vi "Autonomous Independent.vi"() -> ()   [LabVIEW 2017]
doc: "This VI is called when autonomous begins, and will automatically be terminated when autonomous ends. You can carry out timed or sensor driven robot movement independently without needing to return to the caller."
uses:
  <vilib>/Rock Robotics/WPI/DriverStation/WPI_DriverStationPositionInfo.ctl
  <vilib>/Rock Robotics/WPI/DriverStation/WPI_DriverStationAllianceInfo.ctl
  Public/Documents/Cross The Road Electronics/Phoenix-LabVIEW/Motor Controller/Controls/CTRE_Phoenix_MotorControl_ControlMode.ctl
  <vilib>/Rock Robotics/Network Tables/NT Read String.vi
  <vilib>/Rock Robotics/Network Tables/NT Read Number.vi
  <vilib>/Rock Robotics/Network Tables/NT Read Numeric Array.vi
  <vilib>/Rock Robotics/Network Tables/NT Read String Array.vi
  Robot Global Data.vi
  <vilib>/Rock Robotics/WPI/Ultrasonic/WPI_SonarMB1010AnalogRefNum Registry Get.vi
  <vilib>/Rock Robotics/WPI/Ultrasonic/WPI_SonarMB1010AnalogGetRange.vi
panel:
  out "Alliance":T1
  out "Position":T2
  out "FMS Data Array":string[](array[string])
  out "Scale":string
  out "Switch":string
  out "Setpoint2":dbl
  out "Setpoint":dbl
  in  "Z Drive PID Gains":T3={"Position"=0.04, "Interval"=0.0, "Derivative"=0.0}
  # "Be sure to right-click and choose Data Operations>>Make Current Value default if you want to save the array values with the VI"
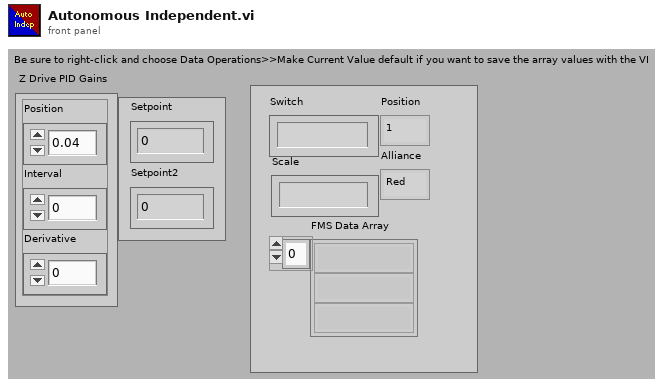
[diagram p1: front panel]
types:
  T1 = typedef "WPI_DriverStationAllianceInfo.ctl" = enum16{"Red", "Blue", "Invalid"}
  T2 = typedef "WPI_DriverStationPositionInfo.ctl" = enum16{"1", "2", "3"}
  T3 = cluster{"Position":dbl, "Interval":dbl, "Derivative":dbl}
  T4 = enum16{"Front Left", "Front Right", "Back Left", "Back Right"}
  T5 = typedef "WPI_SonarMB1010AnalogDeviceRef.ctl" = cluster{"AIDeviceRef":T6, "Scaling factor (V/in)":dbl, "Average Bits":u8}
  T6 = typedef "WPI_AnalogChannelDevRef.ctl" = cluster{"DevStatus":errorcluster, "Analog Channel":T7}
  T7 = typedef "FPGA_AIChannel.ctl" = enum8{"AI 0", "AI 1", "AI 2", "AI 3", "AI MXP 0", "AI MXP 1", "AI MXP 2", "AI MXP 3", "Invalid"}
  T8 = typedef "WPI_AccelerometerDevRef.ctl" = cluster{"DevStatus":errorcluster, "Scaling":T9, "Analog Channels":T10, "I2C Bus":T11, "SPI Bus":T12, "Accel Range":T13, "ADXL Axes":T14, "Handle":i32, "Device Address":u8, "Accel Type":enum16{"Analog", "ADXL345 I2C", "ADXL345 SPI", "Internal", "ADXL362 SPI"}}
  T9 = typedef "WPI_AccelerometerScaling.ctl" = cluster{"Gain (VoltsPerG)":dbl, "Center Voltage":dbl}
  T10 = typedef "WPI_AccelerometerAnalogChannels.ctl" = cluster{"X-Axis":T7, "Y-Axis":T7, "Z-Axis":T7}
  T11 = typedef "i2c_bus.ctl" = enum16{"I2C On-Board", "I2C MXP", "Invalid"}
  T12 = typedef "spi_bus.ctl" = enum16{"SPI On-Board, CS0", "SPI On-Board, CS1", "SPI On-Board, CS2", "SPI On-Board, CS3", "SPI MXP", "Invalid"}
  T13 = typedef "ADXL345 Range.ctl" = u8
  T14 = typedef "WPI_AccelerometerADXL345 Axes.ctl" = cluster{"X-Axis":bool, "Y-Axis":bool, "Z-Axis":bool}
  T15 = cluster{"X-Axis":dbl, "Y-Axis":dbl, "Z-Axis":dbl}
  T16 = typedef "WPI_EncoderDevRef.ctl" = cluster{"DevStatus":errorcluster, "EncoderIndex":T17, "CounterIndex":T18, "DistancePerCount":dbl, "Decoding Type":T19}
  T17 = typedef "FPGA_EncoderIdx.ctl" = enum8{"Enc 0", "Enc 1", "Enc 2", "Enc 3", "Enc 4", "Enc 5", "Enc 6", "Enc 7", "Invalid"}
  T18 = typedef "FPGA_CounterCtrSystemIndex.ctl" = enum8{"Ctr 0", "Ctr 1", "Ctr 2", "Ctr 3", "Ctr 4", "Ctr 5", "Ctr 6", "Ctr 7", "Invalid"}
  T19 = typedef "WPI_EncoderType.ctl" = enum16{"1x", "2x", "4x"}
  T20 = typedef "WPI_MotorControlDeviceRef.ctl" = cluster{"DeviceStatus":errorcluster, "Type":T21, "PWM":cluster{"PWM Channel":T22, "DeadBand":T23}, "CAN":cluster{"Device Number":u8, "SetOutput VI Ref":variant, "GetOutput VI Ref":variant, "Enable VI Ref":variant, "Disable VI Ref":variant, "Data":variant}, "Invert":bool, "DIO PWM":cluster{"PWM \"Enable\" Channel":T22, "DIOChannel":T24, "PWM Rate":dbl}}
  T21 = typedef "WPI_MotorControlType.ctl" = enum16{"PWM", "CAN", "DIO PWM"}
  T22 = typedef "FPGA_DIOPWMChannel.ctl" = enum8{"PWM 0", "PWM 1", "PWM 2", "PWM 3", "PWM 4", "PWM 5", "PWM 6", "PWM 7", "PWM 8", "PWM 9", "PWM MXP 0", "PWM MXP 1", "PWM MXP 2", "PWM MXP 3", "PWM MXP 4", "PWM MXP 5", "PWM MXP 6", "PWM MXP 7", "PWM MXP 8", "PWM MXP 9", "Invalid"}
  T23 = typedef "WPI_PWMDeadband.ctl" = cluster{"Name":string, "maxPositivePwm":i32, "minPositivePwm":i32, "centerPwm":i32, "maxNegativePwm":i32, "minNegativePwm":i32, "angularRange":u16}
  T24 = typedef "FPGA_DIOChannel.ctl" = enum8{"DIO 0", "DIO 1", "DIO 2", "DIO 3", "DIO 4", "DIO 5", "DIO 6", "DIO 7", "DIO 8", "DIO 9", "DIO MXP 0", "DIO MXP 1", "DIO MXP 2", "DIO MXP 3", "DIO MXP 4", "DIO MXP 5", "DIO MXP 6", "DIO MXP 7", "DIO MXP 8", "DIO MXP 9", "DIO MXP 10", "DIO MXP 11", "DIO MXP 12", "DIO MXP 13", "DIO MXP 14", "DIO MXP 15", "SPI Port CS1", "SPI Port CS2", "SPI Port CS3", "SPI Port MISO", "SPI Port MOSI", "Invalid"}
  T25 = typedef "CTRE_Phoenix_MotorControl_ControlMode.ctl" = u16
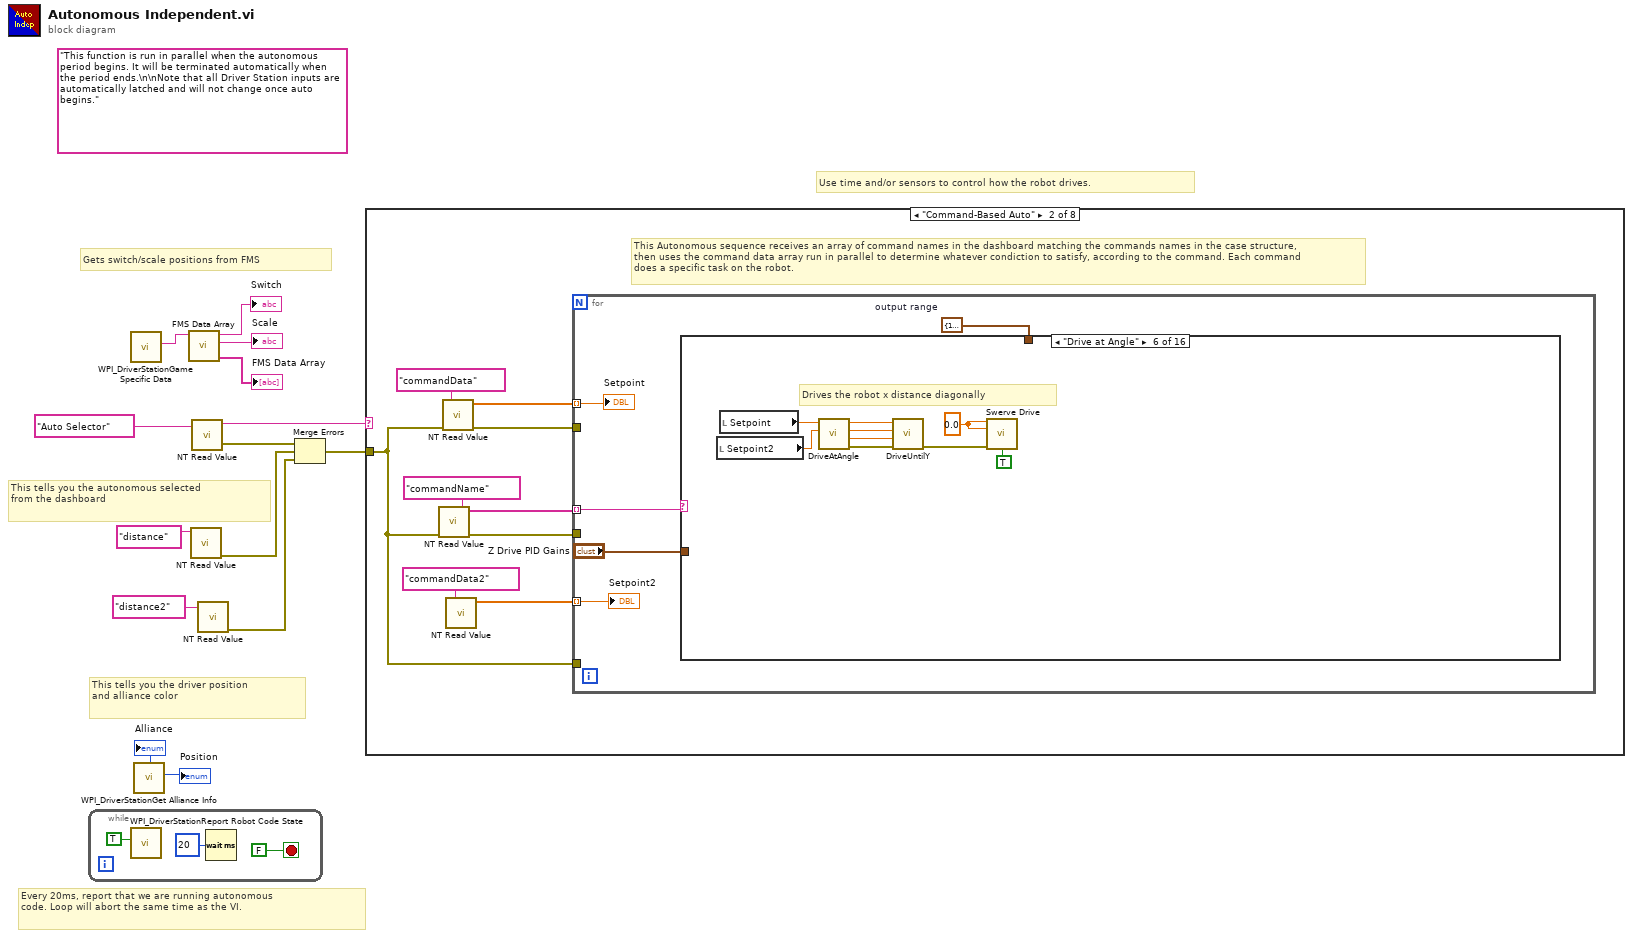
[diagram p0: block diagram]
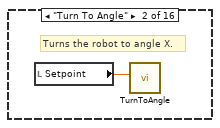
[diagram p4: hidden frame]
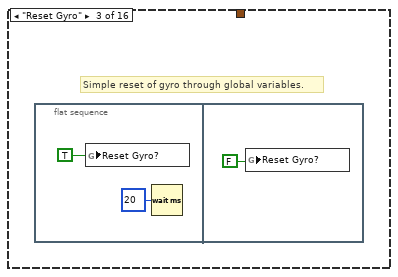
[diagram p5: hidden frame]
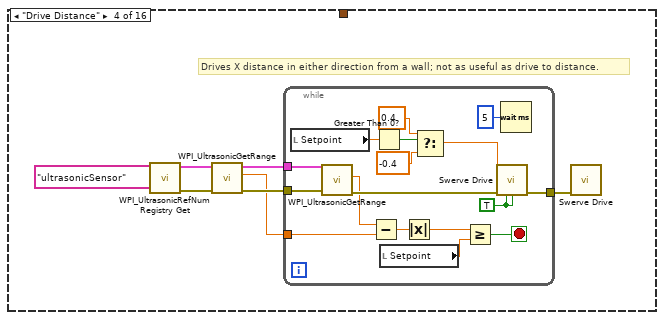
[diagram p6: hidden frame]
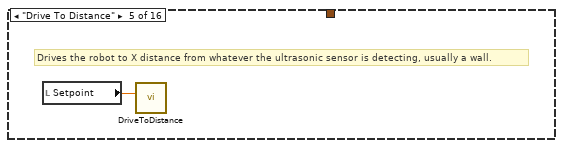
[diagram p7: hidden frame]
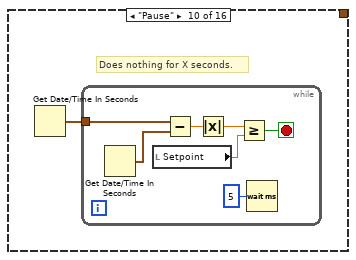
[diagram p11: hidden frame]
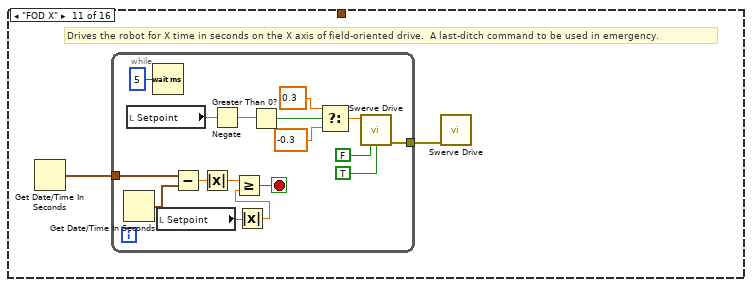
[diagram p12: hidden frame]
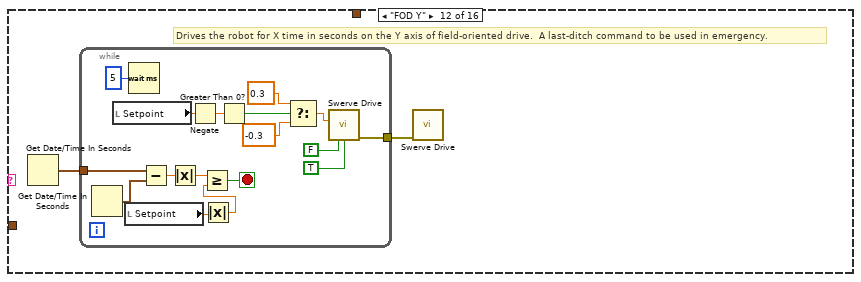
[diagram p13: hidden frame]
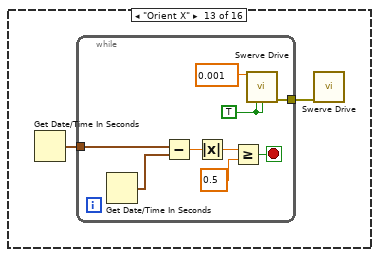
[diagram p14: hidden frame]
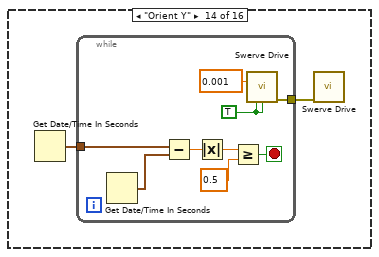
[diagram p15: hidden frame]
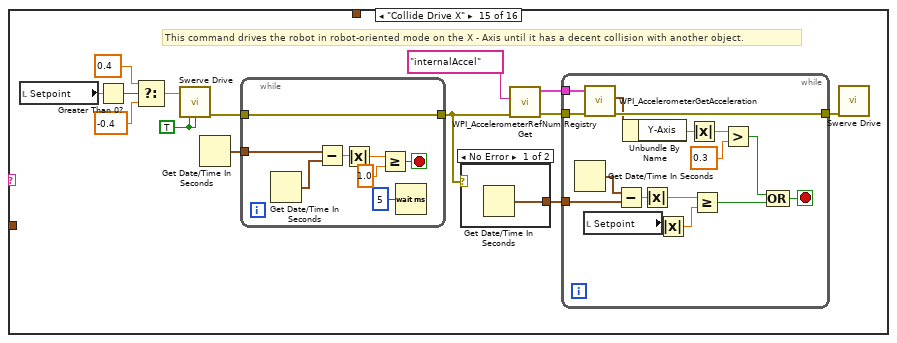
[diagram p16: hidden frame]
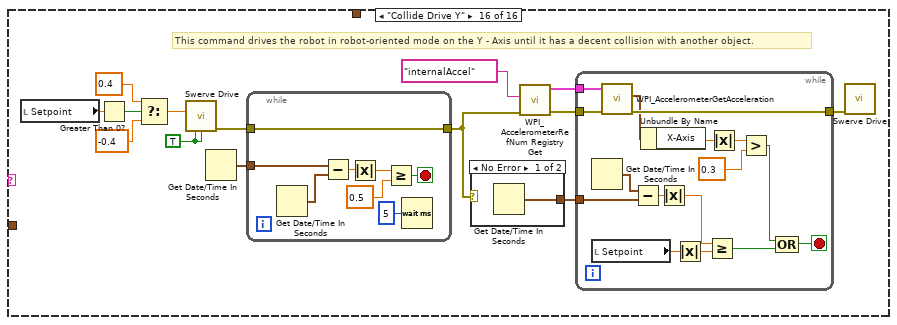
[diagram p18: hidden frame]
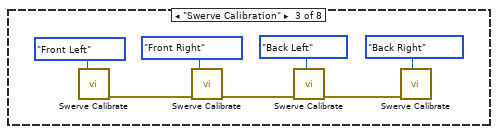
[diagram p20: hidden frame]
diagram:
  (unwired) "This function is run in parallel when the autonomous period begins. It will be terminated automatically when the period ends.\n\nNote that all Driver Station inputs are automatically latched and will not change once auto begins."
  # "Gets switch/scale positions from FMS"
  # "This tells you the autonomous selected\nfrom the dashboard"
  # "Every 20ms, report that we are running autonomous\ncode. Loop will abort the same time as the VI."
  # "Use time and/or sensors to control how the robot drives."
  # "This tells you the driver position\nand alliance color"
  n1 = while {
    stop <- FALSE stop-if-true
    n2 = call <vilib>:"WPI_DriverStationReport Robot Code State.vi"("Autonomous"=TRUE) -> ()  [unwired: 10 in, 1 out]
    n3 = Wait (ms)(milliseconds to wait=u32 20) -> ()  [unwired: 1 out]
  }
  n4 = call <vilib>:"WPI_DriverStationGame Specific Data.vi"() -> ("Game Specific Data"=w6:string)  [unwired: 11 in]
  n5 = call <vilib>:"WPI_DriverStationGet Alliance Info.vi"() -> ("Position"=→"Position":T2, "Alliance"=→"Alliance":T1)  [unwired: 10 out]
  n6 = call "FMS Data Array.vi"("Game Data"=w6) -> ("FMS Data Array"=→"FMS Data Array":string[], "Scale"=→"Scale":string, "Switch"=→"Switch":string)  [unwired: 8 in]
  n7 = call-poly <vilib>:"NT Read Value.vi"("Name"="distance") -> ("error out"=w10:errorcluster)  [unwired: 9 in, 1 out]
  n8 = call-poly <vilib>:"NT Read Value.vi"("Name"="Auto Selector") -> ("error out"=w11:errorcluster, "String"=w13:string)  [unwired: 9 in]
  n9 = call-poly <vilib>:"NT Read Value.vi"("Name"="distance2") -> ("error out"=w8:errorcluster)  [unwired: 9 in, 1 out]
  n10 = Merge Errors(w11, w10, w8) -> (w9:errorcluster)
  n11 = case shown="\"Command-Based Auto\"" w13 {
    tunnel: w9 -> [_ w20 _ _ _ _ _ _]
    frame Default {
      # "You can put your main auto here, or you can right-click on the case and make any\nother frame be the default case."
      # "This is the frame that will execute if no selection is made, or if it is not recognized"
    }
    frame "Command-Based Auto" {
      # "This Autonomous sequence receives an array of command names in the dashboard matching the commands names in the case structure, \nthen uses the command data array run in parallel to determine whatever condiction to satisfy, according to the command. Each command\ndoes a specific task on the robot."
      n12 = call-poly <vilib>:"NT Read Value.vi"("error in"=w20, "Name"="commandName") -> ("error out"=w21:errorcluster, "String Array"=w24:string[])  [unwired: 8 in]
      n13 = call-poly <vilib>:"NT Read Value.vi"("error in"=w20, "Name"="commandData") -> ("error out"=w22:errorcluster, "Numeric Array"=w23:dbl[])  [unwired: 8 in]
      n14 = call-poly <vilib>:"NT Read Value.vi"("Name"="commandData2") -> ("Numeric Array"=w18:dbl[])  [unwired: 9 in, 1 out]
      n15 = for {
        tunnel: w24 -> [w31] mode=indexing
        tunnel: w23 -> [w28] mode=indexing
        tunnel: w22 -> [_]
        tunnel: w21 -> [_]
        tunnel: w20 -> [_]
        tunnel: w18 -> [w27] mode=indexing
        w29 = cluster{"output high":dbl, "output low":dbl} {"output high"=1.0, "output low"=-1.0}  # output range
        n16 = case shown="\"Drive at Angle\"" w31 {
          tunnel: "Z Drive PID Gains" -> [_ _ _ _ _ _ _ _ _ _ _ _ _ _ _ _]
          tunnel: w29 -> [_ _ _ _ _ _ _ _ _ _ _ _ _ _ _ _]
          frame Default {
          }
          frame "Turn To Angle" {
            # "Turns the robot to angle X."
            n17 = local read "Setpoint"() -> (w32:dbl)
            n18 = call "TurnToAngle.vi"("Target Angle"=w32) -> ()  [unwired: 10 in, 1 out]
          }
          frame "Reset Gyro" {
            # "Simple reset of gyro through global variables."
            n19 = flat-sequence {
              frame #0 {
                n20 = global write "Robot Global Data.vi" "Reset Gyro?"(TRUE ("Reset Gyro?")) -> ()
                n21 = Wait (ms)(milliseconds to wait=u32 20) -> ()  [unwired: 1 out]
              }
              frame #1 {
                n22 = global write "Robot Global Data.vi" "Reset Gyro?"(FALSE ("Reset Gyro?")) -> ()
              }
            }
          }
          frame "Drive Distance" {
            # "Drives X distance in either direction from a wall; not as useful as drive to distance."
            n23 = call-poly <vilib>:"WPI_UltrasonicRefNum Registry Get.vi"("refnum name"="ultrasonicSensor") -> ("error out"=w38:errorcluster, "SonarMB1010AnalogDevRef"=w40:T5)  [unwired: 9 in]
            n24 = call-poly <vilib>:"WPI_UltrasonicGetRange.vi"("error in"=w38, "SonarMB1010AnalogDevRef"=w40) -> ("error out"=w37:errorcluster, "Distance"=w36:dbl, "SonarMB1010AnalogDevRef"=w39:T5)  [unwired: 7 in]
            n25 = while {
              tunnel: [w58] -> w41
              tunnel: w36 -> [w53]
              tunnel: w39 -> [w56]
              tunnel: w37 -> [w55]
              stop <- w57 stop-if-true
              w48 = TRUE ("Robot Centric?")
              n26 = local read "Setpoint"() -> (w46:dbl)
              n27 = call-poly <vilib>:"WPI_UltrasonicGetRange.vi"("error in"=w55, "SonarMB1010AnalogDevRef"=w56) -> ("error out"=w54:errorcluster, "Distance"=w47:dbl)  [unwired: 7 in, 1 out]
              n28 = Subtract(x=w47, y=w53) -> (x-y=w44:dbl)
              n29 = Greater Than 0?(x=w46) -> (x > 0?=w49:bool)
              n30 = local read "Setpoint"() -> (w45:dbl)
              n31 = Absolute Value(x=w44) -> (abs(x)=w59:dbl)
              n32 = Select(t=0.4 ("Y"), s=w49, f=-0.4 ("Y")) -> (s? t:f=w52:dbl)
              n33 = Greater Or Equal?(x=w59, y=w45) -> (x >= y?=w57:bool)
              n34 = call "Swerve Drive.vi"("Y"=w52, "Error In"=w54, "Robot Centric?"=w48, "Autonomous?"=w48) -> ("Error Out"=w58:errorcluster)  [unwired: 7 in, 4 out]
              n35 = Wait (ms)(milliseconds to wait=u32 5) -> ()  [unwired: 1 out]
            }
            n36 = call "Swerve Drive.vi"("Error In"=w41) -> ()  [unwired: 10 in, 5 out]
          }
          frame "Drive To Distance" {
            # "Drives the robot to X distance from whatever the ultrasonic sensor is detecting, usually a wall."
            n37 = local read "Setpoint"() -> (w60:dbl)
            n38 = call "DriveToDistance.vi"("Setpoint"=w60) -> ()  [unwired: 10 in, 1 out]
          }
          frame "Drive at Angle" {
            w63 = 0.0 ("Y")
            # "Drives the robot x distance diagonally"
            n39 = local read "Setpoint2"() -> (w61:dbl)
            n40 = local read "Setpoint"() -> (w62:dbl)
            n41 = call "DriveAtAngle.vi"("Target Angle"=w62, "Distance"=w61) -> ("y-axis distance"=w68:dbl, "x"=w67:dbl, "y"=w66:dbl, "Error Out"=w69:errorcluster)  [unwired: 5 in]
            n42 = call "DriveUntilY.vi"("error in"=w69, "y"=w66, "x"=w67, "y-axis distance"=w68) -> ("error out"=w65:errorcluster)  [unwired: 7 in]
            n43 = call "Swerve Drive.vi"("X"=w63, "Y"=w63, "Error In"=w65, "Autonomous?"=TRUE) -> ()  [unwired: 7 in, 5 out]
          }
          frame "Lift Main" {
          }
          frame "Drive Until Distance" {
          }
          frame "Side Compare" {
          }
          frame "Pause" {
            # "Does nothing for X seconds."
            n44 = Get Date/Time In Seconds() -> (seconds since 1Jan1904=w70:timestamp)
            n45 = while {
              tunnel: w70 -> [w77]
              stop <- w72 stop-if-true
              n46 = Get Date/Time In Seconds() -> (seconds since 1Jan1904=w76:timestamp)
              n47 = local read "Setpoint"() -> (w73:dbl)
              n48 = Subtract(x=w77, y=w76) -> (x-y=w75:dbl)
              n49 = Absolute Value(x=w75) -> (abs(x)=w74:dbl)
              n50 = Greater Or Equal?(x=w74, y=w73) -> (x >= y?=w72:bool)
              n51 = Wait (ms)(milliseconds to wait=u32 5) -> ()  [unwired: 1 out]
            }
          }
          frame "FOD X" {
            # "Drives the robot for X time in seconds on the X axis of field-oriented drive.  A last-ditch command to be used in emergency."
            n52 = Get Date/Time In Seconds() -> (seconds since 1Jan1904=w79:timestamp)
            n53 = while {
              tunnel: w79 -> [w96]
              tunnel: [w90] -> w78
              stop <- w91 stop-if-true
              n54 = Get Date/Time In Seconds() -> (seconds since 1Jan1904=w95:timestamp)
              n55 = local read "Setpoint"() -> (w83:dbl)
              n56 = Wait (ms)(milliseconds to wait=u32 5) -> ()  [unwired: 1 out]
              n57 = local read "Setpoint"() -> (w92:dbl)
              n58 = Subtract(x=w96, y=w95) -> (x-y=w94:dbl)
              n59 = Absolute Value(x=w94) -> (abs(x)=w93:dbl)
              n60 = Negate(x=w83) -> (-x=w80:dbl)
              n61 = Absolute Value(x=w92) -> (abs(x)=w81:dbl)
              n62 = Greater Or Equal?(x=w93, y=w81) -> (x >= y?=w91:bool)
              n63 = Greater Than 0?(x=w80) -> (x > 0?=w84:bool)
              n64 = Select(t=0.3 ("X"), s=w84, f=-0.3 ("X")) -> (s? t:f=w85:dbl)
              n65 = call "Swerve Drive.vi"("X"=w85, "Robot Centric?"=FALSE, "Autonomous?"=TRUE) -> ("Error Out"=w90:errorcluster)  [unwired: 8 in, 4 out]
            }
            n66 = call "Swerve Drive.vi"("Error In"=w78) -> ()  [unwired: 10 in, 5 out]
          }
          frame "FOD Y" {
            # "Drives the robot for X time in seconds on the Y axis of field-oriented drive.  A last-ditch command to be used in emergency."
            n67 = Get Date/Time In Seconds() -> (seconds since 1Jan1904=w98:timestamp)
            n68 = while {
              tunnel: w98 -> [w115]
              tunnel: [w109] -> w97
              stop <- w110 stop-if-true
              n69 = Get Date/Time In Seconds() -> (seconds since 1Jan1904=w114:timestamp)
              n70 = local read "Setpoint"() -> (w102:dbl)
              n71 = local read "Setpoint"() -> (w111:dbl)
              n72 = Wait (ms)(milliseconds to wait=u32 5) -> ()  [unwired: 1 out]
              n73 = Subtract(x=w115, y=w114) -> (x-y=w113:dbl)
              n74 = Absolute Value(x=w113) -> (abs(x)=w112:dbl)
              n75 = Negate(x=w102) -> (-x=w99:dbl)
              n76 = Absolute Value(x=w111) -> (abs(x)=w100:dbl)
              n77 = Greater Or Equal?(x=w112, y=w100) -> (x >= y?=w110:bool)
              n78 = Greater Than 0?(x=w99) -> (x > 0?=w104:bool)
              n79 = Select(t=0.3 ("X"), s=w104, f=-0.3 ("X")) -> (s? t:f=w103:dbl)
              n80 = call "Swerve Drive.vi"("Y"=w103, "Robot Centric?"=FALSE, "Autonomous?"=TRUE) -> ("Error Out"=w109:errorcluster)  [unwired: 8 in, 4 out]
            }
            n81 = call "Swerve Drive.vi"("Error In"=w97) -> ()  [unwired: 10 in, 5 out]
          }
          frame "Orient X" {
            n82 = Get Date/Time In Seconds() -> (seconds since 1Jan1904=w117:timestamp)
            n83 = while {
              tunnel: w117 -> [w126]
              tunnel: [w120] -> w116
              stop <- w119 stop-if-true
              w121 = TRUE ("Robot Centric?")
              n84 = Get Date/Time In Seconds() -> (seconds since 1Jan1904=w125:timestamp)
              n85 = Subtract(x=w126, y=w125) -> (x-y=w124:dbl)
              n86 = Absolute Value(x=w124) -> (abs(x)=w123:dbl)
              n87 = Greater Or Equal?(x=w123, y=0.5) -> (x >= y?=w119:bool)
              n88 = call "Swerve Drive.vi"("X"=0.001 ("Y"), "Robot Centric?"=w121, "Autonomous?"=w121) -> ("Error Out"=w120:errorcluster)  [unwired: 8 in, 4 out]
            }
            n89 = call "Swerve Drive.vi"("Error In"=w116) -> ()  [unwired: 10 in, 5 out]
          }
          frame "Orient Y" {
            n90 = Get Date/Time In Seconds() -> (seconds since 1Jan1904=w128:timestamp)
            n91 = while {
              tunnel: w128 -> [w137]
              tunnel: [w130] -> w127
              stop <- w129 stop-if-true
              w132 = TRUE ("Robot Centric?")
              n92 = Get Date/Time In Seconds() -> (seconds since 1Jan1904=w136:timestamp)
              n93 = Subtract(x=w137, y=w136) -> (x-y=w135:dbl)
              n94 = Absolute Value(x=w135) -> (abs(x)=w134:dbl)
              n95 = Greater Or Equal?(x=w134, y=0.5) -> (x >= y?=w129:bool)
              n96 = call "Swerve Drive.vi"("Y"=0.001, "Robot Centric?"=w132, "Autonomous?"=w132) -> ("Error Out"=w130:errorcluster)  [unwired: 8 in, 4 out]
            }
            n97 = call "Swerve Drive.vi"("Error In"=w127) -> ()  [unwired: 10 in, 5 out]
          }
          frame "Collide Drive X" {
            w146 = TRUE ("Robot Centric?")
            # "This command drives the robot in robot-oriented mode on the X - Axis until it has a decent collision with another object."
            n98 = local read "Setpoint"() -> (w151:dbl)
            n99 = Greater Than 0?(x=w151) -> (x > 0?=w150:bool)
            n100 = Select(t=0.4, s=w150, f=-0.4) -> (s? t:f=w147:dbl)
            n101 = call "Swerve Drive.vi"("X"=w147, "Robot Centric?"=w146, "Autonomous?"=w146) -> ("Error Out"=w145:errorcluster)  [unwired: 8 in, 4 out]
            n102 = Get Date/Time In Seconds() -> (seconds since 1Jan1904=w144:timestamp)
            n103 = while {
              tunnel: w145 -> [w169]
              tunnel: w144 -> [w176]
              tunnel: [w169] -> w139
              stop <- w170 stop-if-true
              n104 = Get Date/Time In Seconds() -> (seconds since 1Jan1904=w175:timestamp)
              n105 = Subtract(x=w176, y=w175) -> (x-y=w174:dbl)
              n106 = Absolute Value(x=w174) -> (abs(x)=w173:dbl)
              n107 = Greater Or Equal?(x=w173, y=1.0) -> (x >= y?=w170:bool)
              n108 = Wait (ms)(milliseconds to wait=u32 5) -> ()  [unwired: 1 out]
            }
            n109 = case shown="No Error" w139 {
              tunnel: [w152 _] -> w138
              frame No Error {
                n110 = Get Date/Time In Seconds() -> (seconds since 1Jan1904=w152:timestamp)
              }
              frame Error {
              }
            }
            n111 = call <vilib>:"WPI_AccelerometerRefNum Registry Get.vi"("error in (no error)"=w139, "refnum name"="internalAccel") -> ("error out"=w142:errorcluster, "AccelerometerDevRef"=w141:T8)  [unwired: 8 in]
            n112 = while {
              tunnel: w142 -> [w168]
              tunnel: w141 -> [w167]
              tunnel: [w166] -> w140
              tunnel: w138 -> [w164]
              stop <- w165 stop-if-true
              n113 = Get Date/Time In Seconds() -> (seconds since 1Jan1904=w163:timestamp)
              n114 = local read "Setpoint"() -> (w159:dbl)
              n115 = call <vilib>:"WPI_AccelerometerGetAcceleration.vi"("error in"=w168, "AccelerometerDevRef"=w167) -> ("error out"=w166:errorcluster, "Accelerations"=w157:T15)  [unwired: 7 in, 1 out]
              n116 = Subtract(x=w163, y=w164) -> (x-y=w162:dbl)
              n117 = Unbundle By Name(w157) -> ("Y-Axis"=w156:dbl)
              n118 = Absolute Value(x=w162) -> (abs(x)=w161:dbl)
              n119 = Absolute Value(x=w159) -> (abs(x)=w158:dbl)
              n120 = Absolute Value(x=w156) -> (abs(x)=w154:dbl)
              n121 = Greater Or Equal?(x=w161, y=w158) -> (x >= y?=w160:bool)
              n122 = Greater?(x=w154, y=0.3) -> (0:w153:bool)
              n123 = Compound Arithmetic op=OR(w153, w160) -> (w165:bool)
            }
            n124 = call "Swerve Drive.vi"("Error In"=w140) -> ()  [unwired: 10 in, 5 out]
          }
          frame "Collide Drive Y" {
            w186 = TRUE ("Robot Centric?")
            # "This command drives the robot in robot-oriented mode on the Y - Axis until it has a decent collision with another object."
            n125 = local read "Setpoint"() -> (w190:dbl)
            n126 = Greater Than 0?(x=w190) -> (x > 0?=w189:bool)
            n127 = Select(t=0.4, s=w189, f=-0.4) -> (s? t:f=w177:dbl)
            n128 = call "Swerve Drive.vi"("Y"=w177, "Robot Centric?"=w186, "Autonomous?"=w186) -> ("Error Out"=w185:errorcluster)  [unwired: 8 in, 4 out]
            n129 = Get Date/Time In Seconds() -> (seconds since 1Jan1904=w184:timestamp)
            n130 = while {
              tunnel: w185 -> [w208]
              tunnel: w184 -> [w215]
              tunnel: [w208] -> w179
              stop <- w209 stop-if-true
              n131 = Get Date/Time In Seconds() -> (seconds since 1Jan1904=w214:timestamp)
              n132 = Subtract(x=w215, y=w214) -> (x-y=w213:dbl)
              n133 = Absolute Value(x=w213) -> (abs(x)=w212:dbl)
              n134 = Greater Or Equal?(x=w212, y=0.5) -> (x >= y?=w209:bool)
              n135 = Wait (ms)(milliseconds to wait=u32 5) -> ()  [unwired: 1 out]
            }
            n136 = case shown="No Error" w179 {
              tunnel: [w191 _] -> w178
              frame No Error {
                n137 = Get Date/Time In Seconds() -> (seconds since 1Jan1904=w191:timestamp)
              }
              frame Error {
              }
            }
            n138 = call <vilib>:"WPI_AccelerometerRefNum Registry Get.vi"("error in (no error)"=w179, "refnum name"="internalAccel") -> ("error out"=w182:errorcluster, "AccelerometerDevRef"=w181:T8)  [unwired: 8 in]
            n139 = while {
              tunnel: w182 -> [w207]
              tunnel: w181 -> [w206]
              tunnel: [w205] -> w180
              tunnel: w178 -> [w202]
              stop <- w204 stop-if-true
              n140 = Get Date/Time In Seconds() -> (seconds since 1Jan1904=w201:timestamp)
              n141 = local read "Setpoint"() -> (w197:dbl)
              n142 = call <vilib>:"WPI_AccelerometerGetAcceleration.vi"("error in"=w207, "AccelerometerDevRef"=w206) -> ("error out"=w205:errorcluster, "Accelerations"=w195:T15)  [unwired: 7 in, 1 out]
              n143 = Subtract(x=w201, y=w202) -> (x-y=w200:dbl)
              n144 = Unbundle By Name(w195) -> ("X-Axis"=w194:dbl)
              n145 = Absolute Value(x=w200) -> (abs(x)=w199:dbl)
              n146 = Absolute Value(x=w197) -> (abs(x)=w196:dbl)
              n147 = Greater Or Equal?(x=w199, y=w196) -> (x >= y?=w198:bool)
              n148 = Absolute Value(x=w194) -> (abs(x)=w193:dbl)
              n149 = Greater?(x=w193, y=0.3) -> (0:w203:bool)
              n150 = Compound Arithmetic op=OR(w203, w198) -> (w204:bool)
            }
            n151 = call "Swerve Drive.vi"("Error In"=w180) -> ()  [unwired: 10 in, 5 out]
          }
        }
        "Setpoint" <- w28
        "Setpoint2" <- w27
      }
    }
    frame "Swerve Calibration" {
      n152 = call "Swerve Calibrate.vi"("Wheel Corner"=T4."Front Left") -> ("error out"=w218:errorcluster)  [unwired: 10 in]
      n153 = call "Swerve Calibrate.vi"("error in (no error)"=w218, "Wheel Corner"=T4."Front Right") -> ("error out"=w217:errorcluster)  [unwired: 9 in]
      n154 = call "Swerve Calibrate.vi"("error in (no error)"=w217, "Wheel Corner"=T4."Back Left") -> ("error out"=w216:errorcluster)  [unwired: 9 in]
      n155 = call "Swerve Calibrate.vi"("error in (no error)"=w216, "Wheel Corner"=T4."Back Right") -> ()  [unwired: 9 in, 1 out]
    }
    frame "Config 1" {
    }
    frame "Config 2" {
    }
    frame "Config 3" {
    }
    frame "Motor Jog Mode" {
    }
    frame "Unwind Motors" {
      n156 = call <vilib>:"WPI_EncoderRefNum Registry Get.vi"("refnum name"="frontRightEnc") -> ("error out"=w249:errorcluster, "EncoderDevRef"=w248:T16)  [unwired: 9 in]
      n157 = call <vilib>:"WPI_EncoderRefNum Registry Get.vi"("refnum name"="frontLeftEnc") -> ("error out"=w256:errorcluster, "EncoderDevRef"=w257:T16)  [unwired: 9 in]
      n158 = call "CTRE_Phoenix_MotorControl_RefNumRegistryGet.vi"("refnum name"="frontLeftRotation") -> ("error out"=w232:errorcluster, "PhoenixMotorControlDevRef"=w233:T20)  [unwired: 9 in]
      n159 = call "CTRE_Phoenix_MotorControl_RefNumRegistryGet.vi"("refnum name"="frontRightRotation") -> ("error out"=w230:errorcluster, "PhoenixMotorControlDevRef"=w231:T20)  [unwired: 9 in]
      n160 = call <vilib>:"WPI_EncoderGet.vi"("error in (no error)"=w249, "EncoderDevRef"=w248) -> ("error out"=w250:errorcluster, "Distance"=w252:dbl, "EncoderDevRef"=w251:T16)  [unwired: 4 in, 3 out]
      n161 = call <vilib>:"WPI_EncoderGet.vi"("error in (no error)"=w256, "EncoderDevRef"=w257) -> ("error out"=w255:errorcluster, "Distance"=w253:dbl, "EncoderDevRef"=w254:T16)  [unwired: 4 in, 3 out]
      n162 = while {
        tunnel: w251 -> [w303]
        tunnel: w250 -> [w302]
        tunnel: w252 -> [w301]
        tunnel: w231 -> [w290]
        tunnel: w230 -> [w292]
        stop <- w296 stop-if-true
        w289 = T25 0 items=["PercentOutput"=0, "Position"=1, "Velocity"=2, "Current"=3, "Follower"=5, "MotionProfile"=6, "MotionMagic"=7, "MotionMagicArc"=8, "MotionProfileArc"=10, "Disabled"=15] ("Control Mode")
        n163 = Greater Than 0?(x=w301) -> (x > 0?=w300:bool)
        n164 = call <vilib>:"WPI_EncoderGet.vi"("error in (no error)"=w302, "EncoderDevRef"=w303) -> ("Distance"=w295:dbl)  [unwired: 4 in, 5 out]
        n165 = Select(t=0.5, s=w300, f=-0.5) -> (s? t:f=w291:dbl)
        n166 = In Range and Coerce(upper limit=1.0, x=w295, lower limit=-1.0) -> (In Range?=w296:bool)  [unwired: 1 out]
        n167 = call "CTRE_Phoenix_MotorControl_Set.vi"("error in (no error)"=w292, "Output"=w291, "Control Mode"=w289, "PhoenixMotorControlDevRef"=w290) -> ()  [unwired: 6 in, 2 out]
        n168 = Wait (ms)(milliseconds to wait=u32 5) -> ()  [unwired: 1 out]
      }
      n169 = while {
        tunnel: w254 -> [w318]
        tunnel: w255 -> [w317]
        tunnel: w253 -> [w316]
        tunnel: w233 -> [w307]
        tunnel: w232 -> [w306]
        stop <- w311 stop-if-true
        w304 = T25 0 items=["PercentOutput"=0, "Position"=1, "Velocity"=2, "Current"=3, "Follower"=5, "MotionProfile"=6, "MotionMagic"=7, "MotionMagicArc"=8, "MotionProfileArc"=10, "Disabled"=15] ("Control Mode")
        n170 = Greater Than 0?(x=w316) -> (x > 0?=w315:bool)
        n171 = call <vilib>:"WPI_EncoderGet.vi"("error in (no error)"=w317, "EncoderDevRef"=w318) -> ("Distance"=w310:dbl)  [unwired: 4 in, 5 out]
        n172 = Select(t=0.5, s=w315, f=-0.5) -> (s? t:f=w305:dbl)
        n173 = In Range and Coerce(upper limit=1.0, x=w310, lower limit=-1.0) -> (In Range?=w311:bool)  [unwired: 1 out]
        n174 = call "CTRE_Phoenix_MotorControl_Set.vi"("error in (no error)"=w306, "Output"=w305, "Control Mode"=w304, "PhoenixMotorControlDevRef"=w307) -> ()  [unwired: 6 in, 2 out]
        n175 = Wait (ms)(milliseconds to wait=u32 5) -> ()  [unwired: 1 out]
      }
      n176 = call <vilib>:"WPI_EncoderRefNum Registry Get.vi"("refnum name"="backRightEnc") -> ("error out"=w237:errorcluster, "EncoderDevRef"=w236:T16)  [unwired: 9 in]
      n177 = call <vilib>:"WPI_EncoderRefNum Registry Get.vi"("refnum name"="backLeftEnc") -> ("error out"=w244:errorcluster, "EncoderDevRef"=w245:T16)  [unwired: 9 in]
      n178 = call "CTRE_Phoenix_MotorControl_RefNumRegistryGet.vi"("refnum name"="backRightRotation") -> ("error out"=w227:errorcluster, "PhoenixMotorControlDevRef"=w228:T20)  [unwired: 9 in]
      n179 = call "CTRE_Phoenix_MotorControl_RefNumRegistryGet.vi"("refnum name"="backLeftRotation") -> ("error out"=w225:errorcluster, "PhoenixMotorControlDevRef"=w224:T20)  [unwired: 9 in]
      n180 = call <vilib>:"WPI_EncoderGet.vi"("error in (no error)"=w237, "EncoderDevRef"=w236) -> ("error out"=w238:errorcluster, "Distance"=w240:dbl, "EncoderDevRef"=w239:T16)  [unwired: 4 in, 3 out]
      n181 = call <vilib>:"WPI_EncoderGet.vi"("error in (no error)"=w244, "EncoderDevRef"=w245) -> ("error out"=w243:errorcluster, "Distance"=w241:dbl, "EncoderDevRef"=w242:T16)  [unwired: 4 in, 3 out]
      n182 = while {
        tunnel: w239 -> [w273]
        tunnel: w238 -> [w272]
        tunnel: w240 -> [w271]
        tunnel: w228 -> [w262]
        tunnel: w227 -> [w260]
        stop <- w266 stop-if-true
        w259 = T25 0 items=["PercentOutput"=0, "Position"=1, "Velocity"=2, "Current"=3, "Follower"=5, "MotionProfile"=6, "MotionMagic"=7, "MotionMagicArc"=8, "MotionProfileArc"=10, "Disabled"=15] ("Control Mode")
        n183 = Greater Than 0?(x=w271) -> (x > 0?=w270:bool)
        n184 = call <vilib>:"WPI_EncoderGet.vi"("error in (no error)"=w272, "EncoderDevRef"=w273) -> ("Distance"=w265:dbl)  [unwired: 4 in, 5 out]
        n185 = Select(t=0.5, s=w270, f=-0.5) -> (s? t:f=w261:dbl)
        n186 = In Range and Coerce(upper limit=1.0, x=w265, lower limit=-1.0) -> (In Range?=w266:bool)  [unwired: 1 out]
        n187 = call "CTRE_Phoenix_MotorControl_Set.vi"("error in (no error)"=w260, "Output"=w261, "Control Mode"=w259, "PhoenixMotorControlDevRef"=w262) -> ()  [unwired: 6 in, 2 out]
        n188 = Wait (ms)(milliseconds to wait=u32 5) -> ()  [unwired: 1 out]
      }
      n189 = while {
        tunnel: w242 -> [w288]
        tunnel: w243 -> [w287]
        tunnel: w241 -> [w286]
        tunnel: w224 -> [w275]
        tunnel: w225 -> [w277]
        stop <- w281 stop-if-true
        w274 = T25 0 items=["PercentOutput"=0, "Position"=1, "Velocity"=2, "Current"=3, "Follower"=5, "MotionProfile"=6, "MotionMagic"=7, "MotionMagicArc"=8, "MotionProfileArc"=10, "Disabled"=15] ("Control Mode")
        n190 = Greater Than 0?(x=w286) -> (x > 0?=w285:bool)
        n191 = call <vilib>:"WPI_EncoderGet.vi"("error in (no error)"=w287, "EncoderDevRef"=w288) -> ("Distance"=w280:dbl)  [unwired: 4 in, 5 out]
        n192 = Select(t=0.5, s=w285, f=-0.5) -> (s? t:f=w276:dbl)
        n193 = In Range and Coerce(upper limit=1.0, x=w280, lower limit=-1.0) -> (In Range?=w281:bool)  [unwired: 1 out]
        n194 = call "CTRE_Phoenix_MotorControl_Set.vi"("error in (no error)"=w277, "Output"=w276, "Control Mode"=w274, "PhoenixMotorControlDevRef"=w275) -> ()  [unwired: 6 in, 2 out]
        n195 = Wait (ms)(milliseconds to wait=u32 5) -> ()  [unwired: 1 out]
      }
    }
  }
